vi "test.vi"() -> ()   [LabVIEW 2018]
panel:
  out "Time":u32
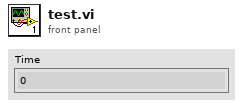
[diagram p1: front panel]
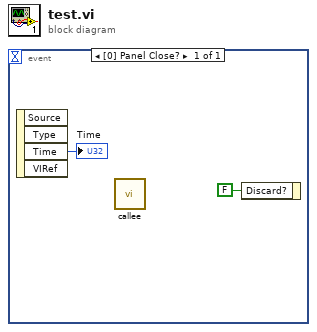
[diagram p0: block diagram]
diagram:
  n1 = event shown="[0] Panel Close?" {
    selector: _ -> [_]
    dyn-events: _ -> [_]
    timeout: _ -> [_]
    event Panel Close? {
      n2 = event-data() -> ("Time"=→"Time":u32)  [unwired: 1 in, 3 out]
      n3 = call "callee.vi"() -> ()  [unwired: 12 in]
      n4 = event-data("Discard?"=FALSE) -> ()  [unwired: 1 in, 1 out]
    }
  }
